vi "SweepConfig.vi"(8 "error in (no error)":errorcluster, 9 "Sweep Time (s)":dbl, 10 "Num Points":u32, 11 "SpecA_ESA in":refnum<class "SpecA_ESA.lvclass">) -> (0 "error out":errorcluster, 3 "SpecA_ESA out":refnum<class "SpecA_ESA.lvclass">)   [LabVIEW 2014, in "SpecA_ESA.lvclass"]
uses:
  SpecA_ESA.lvclass
  SpecA_ESA.lvclass/SpecA_ESA.ctl
  <instrlib>/Agilent ESA PSA Series/Agilent ESA PSA Series.lvlib
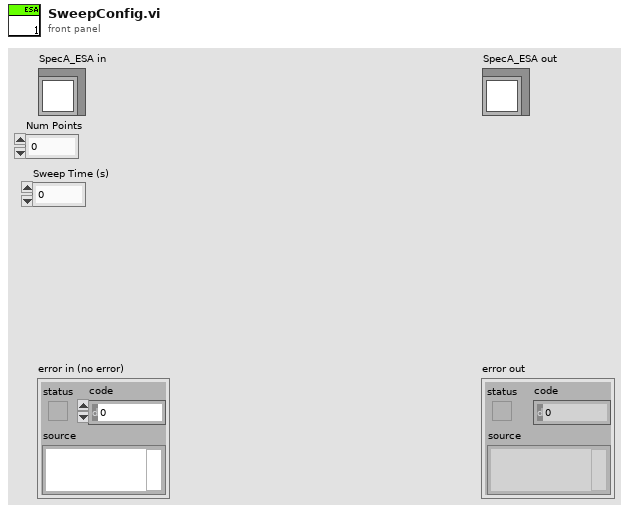
[diagram p1: front panel]
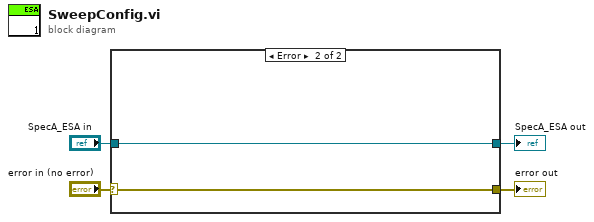
[diagram p0: block diagram]
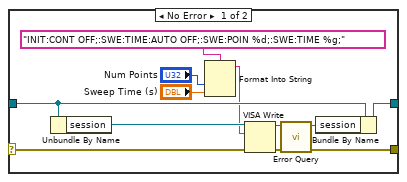
[diagram p2: hidden frame]
diagram:
  n1 = case shown="Error" "error in (no error)" {
    selector: "error in (no error)" -> [w7 w17]
    tunnel: "SpecA_ESA in" -> [w16 w18]
    tunnel: [w15 w18] -> w2
    tunnel: [w5 w17] -> w1
    frame No Error {
      n2 = Unbundle By Name(w16) -> ("session"=w13:refnum<visa-resource-name>)
      n3 = Format Into String(format string="INIT:CONT OFF;:SWE:TIME:AUTO OFF;:SWE:POIN %d;:SWE:TIME %g;", "Num Points", "Sweep Time (s)") -> (resulting string=w10:string)  [unwired: 2 in, 1 out]
      n4 = VISA Write(VISA resource name=w13, write buffer=w10, error in (no error)=w7) -> (VISA resource name out=w14:refnum<visa-resource-name>, error out=w6:errorcluster)  [unwired: 1 out]
      n5 = call <instrlib>:"Error Query.vi"("error in (no error)"=w6, "VISA resource name"=w14) -> ("error out"=w5:errorcluster, "VISA resource name out"=w11:refnum<visa-resource-name>)  [unwired: 6 in, 2 out]
      n6 = Bundle By Name(cluster=w16, "session"=w11) -> (w15:refnum<class "SpecA_ESA.lvclass">)
    }
    frame Error {
    }
  }
  "error out" <- w1
  "SpecA_ESA out" <- w2
